vi "ConvertPB_AOupdates.vi"(0 "PB VLIW Array in":T2(array[cluster]) {"Output Bits" format="%x"}, 1 "Definitions":T1={"External MemorySize"=32768, "Internal Memory Size"=512, "Overhead Ticks"=3, "Min Delay Loops"=3, "Loop Count Correction"=1, "Long Delay Loop Count Correction"=2, "Min Instruction Ticks"=6, "Long Delay Ticks"=4294967295, "Clock Period (s)"=1e-08, "Overhead Time (s)"=3e-08, "Min Instruction Cycle Time (s)"=9e-08, "Long Delay Time (s) "=42.94967298} {"Long Delay Time (s)" format="%.8p"; "Min Instruction Cycle Time (s)" format="%.0p"; "Overhead Time (s)" format="%.0p"; "Clock Period (s)" format="%.0p"; "Long Delay Ticks" format="%.0x"}, 2 "error in (no error)":errorcluster, 3 "Full trigger mask":u32 format="%x") -> (5 "PB VLIW Array out":T2(array[cluster]) {"Output Bits" format="%x"}, 6 "error out":errorcluster)   [LabVIEW 2013, in "PulseBlaster.lvlib"]
doc: "Convert AO updates to two pulses to allow consecutive AO pulses. Replicates the whole PB sequence execpt for channel 22 (AO tigger) and the PB halt channel."
uses:
  PulseBlaster.lvlib
panel:
  in  "BeginLoop pointer":u32
  # "(Period*Long D Ticks)+Overhead time"
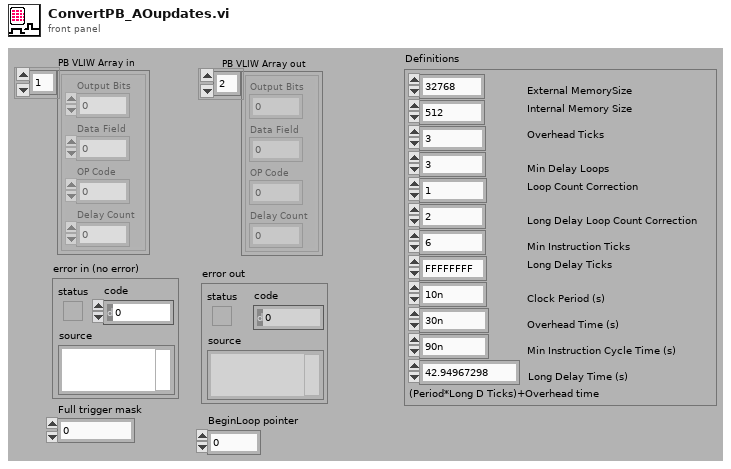
[diagram p1: front panel]
types:
  T1 = cluster{"External MemorySize":u16, "Internal Memory Size":u16, "Overhead Ticks":u8, "Min Delay Loops":u8, "Loop Count Correction":u8, "Long Delay Loop Count Correction":u8, "Min Instruction Ticks":u8, "Long Delay Ticks":u64, "Clock Period (s)":dbl, "Overhead Time (s)":dbl, "Min Instruction Cycle Time (s)":dbl, "Long Delay Time (s) ":dbl}
  T2 = cluster{"Output Bits":u32, "Data Field":u32, "OP Code":u8, "Delay Count":u64}[]
  T3 = cluster{"Output Bits":u32, "Data Field":u32, "OP Code":u8, "Delay Count":u32}[]
  T4 = cluster{"Output Bits":u32, "Data Field":u32, "OP Code":u8, "Delay Count":u64}
  T5 = cluster{"Output Bits":u32, "Data Field":u32, "OP Code":i32, "Delay Count":u64}[]
  T6 = cluster{"Output Bits":u32, "Data Field":u32, "OP Code":u8, u64}
  T7 = cluster{"Output Bits":u32, "BeginLoop pointer":u32, "OP Code":u8, "Delay Count":u64}
  T8 = cluster{"Output Bits":u32, "BeginLoop pointer":u32, "OP Code":i32, "Delay Count":u64}[]
  T9 = cluster{u32, "BeginLoop pointer":u32, "OP Code":u8, u64}
  T10 = cluster{"Output Bits":u32, "Data Field":u32, i32, u64}
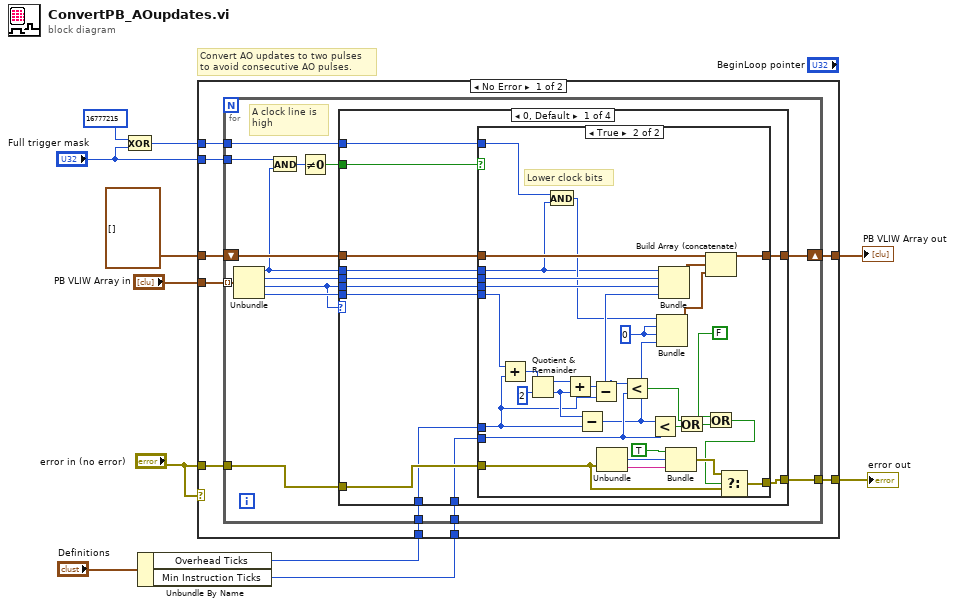
[diagram p0: block diagram]
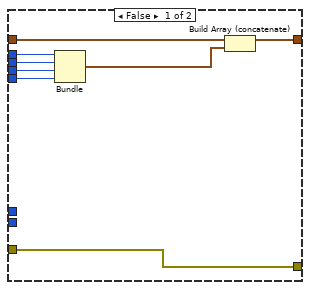
[diagram p2: hidden frame]
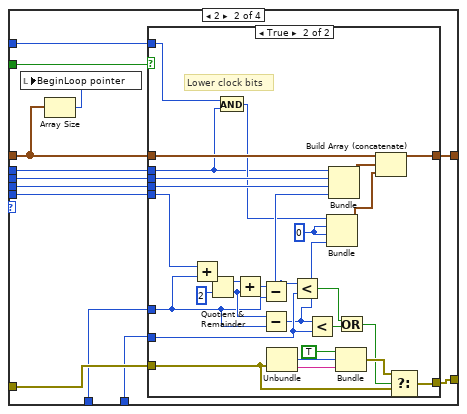
[diagram p3: hidden frame]
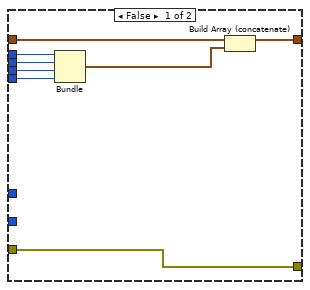
[diagram p4: hidden frame]
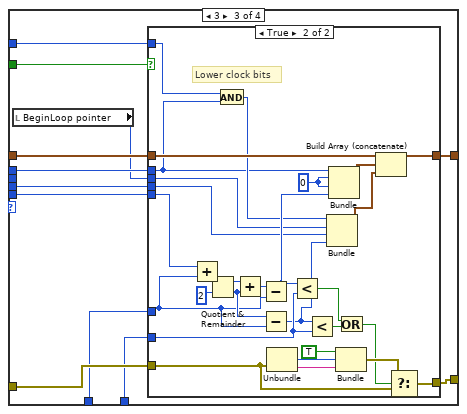
[diagram p5: hidden frame]
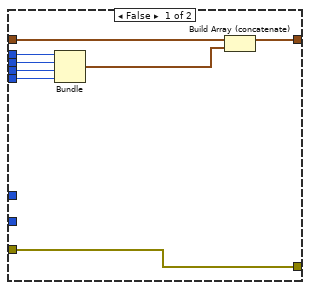
[diagram p6: hidden frame]
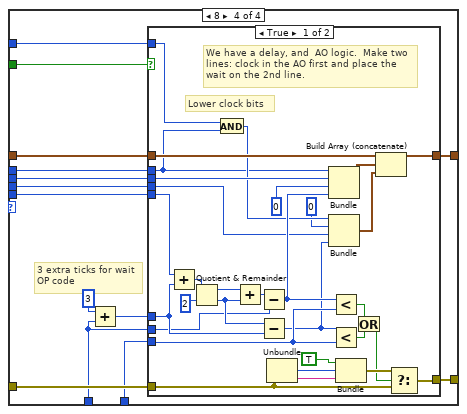
[diagram p7: hidden frame]
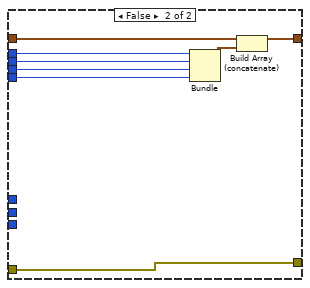
[diagram p8: hidden frame]
diagram:
  # "Convert AO updates to two pulses\nto avoid consecutive AO pulses."
  n1 = Exclusive Or(1:"Full trigger mask", 2:u32 16777215) -> (0:w4:u32)
  n2 = Unbundle By Name("Definitions") -> ("Overhead Ticks"=w2:u8, "Min Instruction Ticks"=w1:u8)
  n3 = case shown="No Error" "error in (no error)" {
    tunnel: T3 [] -> [w20 _]
    tunnel: [w19 w240] -> w10
    tunnel: w2 -> [w18 _]
    tunnel: w1 -> [w17 _]
    tunnel: "PB VLIW Array in" -> [w16 w240]
    tunnel: "error in (no error)" -> [w15 w239]
    tunnel: [w14 w239] -> w8
    tunnel: "Full trigger mask" -> [w13 _]
    tunnel: w4 -> [w12 _]
    frame No Error {
      n4 = for {
        tunnel: w16 -> [w35] mode=indexing
        shift-right: [w27] -> w19
        shift-left: w20 -> [w32]
        tunnel: w15 -> [w31]
        tunnel: [w30] -> w14
        tunnel: w18 -> [w29]
        tunnel: w17 -> [w28]
        tunnel: w13 -> [w22]
        tunnel: w12 -> [w21]
        # "A clock line is \nhigh"
        n5 = Unbundle(w35) -> ("Output Bits"=w25:u32, "Data Field"=w34:u32, "OP Code"=w26:u8, "Delay Count"=w33:u64)
        n6 = And(x=w22, y=w25) -> (x .and. y?=w24:u32)
        n7 = Not Equal To 0?(x=w24) -> (x != 0?=w23:bool)
        n8 = case shown="0, Default" w26 {
          tunnel: w34 -> [w47 w99 _ w199]
          tunnel: w26 -> [w46 w98 w148 w198]
          tunnel: w33 -> [w45 w97 w147 w197]
          tunnel: w32 -> [w44 w89 w140 w196]
          tunnel: w31 -> [w43 w96 w146 w195]
          tunnel: [w42 w95 w145 w194] -> w30
          tunnel: w29 -> [w41 w94 w144 w187]
          tunnel: w28 -> [w40 w93 w143 w193]
          tunnel: w25 -> [w39 w92 w142 w192]
          tunnel: [w38 w91 w141 w191] -> w27
          tunnel: w23 -> [w37 w88 w138 w190]
          tunnel: w21 -> [w36 w87 w137 w186]
          frame 0, Default {
            n9 = case shown="True" w37 {
              tunnel: w39 -> [w55 w57]
              tunnel: w47 -> [w54 w76]
              tunnel: w46 -> [w53 w65]
              tunnel: w45 -> [w52 w86]
              tunnel: [w50 w79] -> w38
              tunnel: w44 -> [w49 w78]
              tunnel: [w48 w71] -> w42
              tunnel: w43 -> [w48 w70]
              tunnel: w41 -> [_ w69]
              tunnel: w40 -> [_ w68]
              tunnel: w36 -> [_ w56]
              frame False {
                n10 = Bundle("Output Bits"=w55, "Data Field"=w54, "OP Code"=w53, "Delay Count"=w52) -> (w51:T4)  [unwired: 1 out]
                n11 = Build Array (concatenate)(w49, w51) -> (w50:T5)
              }
              frame True {
                w58 = 0
                # "Lower clock bits"
                n12 = Add(x=w86, y=w69) -> (x+y=w85:u64)
                n13 = Quotient & Remainder(x=w85, y=u32 2) -> (x-y*floor(x/y)=w83:u64, floor(x/y)=w81:u64)
                n14 = And(x=w56, y=w57) -> (x .and. y?=w64:u32)
                n15 = Add(x=w83, y=w81) -> (x+y=w82:u64)
                n16 = Subtract(x=w81, y=w69) -> (x-y=w66:u64)
                n17 = Subtract(x=w82, y=w69) -> (x-y=w77:u64)
                n18 = Unbundle(w70) -> ("code"=w73:i32, "source"=w74:string)  [unwired: 1 out]
                n19 = Less?(x=w77, y=w68) -> (x < y?=w80:bool)
                n20 = Less?(x=w66, y=w68) -> (x < y?=w67:bool)
                n21 = Bundle(w64, w58, w58, w66) -> (w59:cluster{u32, i32, i32, u64})  [unwired: 1 out]
                n22 = Bundle("Output Bits"=w57, "Data Field"=w76, "OP Code"=w65, w77) -> (w60:T6)  [unwired: 1 out]
                n23 = Bundle(TRUE, "code"=w73, "source"=w74) -> (w72:cluster{bool, "code":i32, "source":string})  [unwired: 1 out]
                n24 = Or(x=w80, y=w67) -> (x .or. y?=w61:bool)
                n25 = Build Array (concatenate)(w78, w60, w59) -> (w79:T5)
                n26 = Or(x=FALSE, y=w61) -> (x .or. y?=w62:bool)
                n27 = Select(t=w72, s=w62, f=w70) -> (s? t:f=w71:errorcluster)
              }
            }
          }
          frame 2 {
            n28 = Array Size(array=w89) -> (size(s)=w90:i32)
            n29 = local write "BeginLoop pointer"(w90) -> ()
            n30 = case shown="True" w88 {
              tunnel: w92 -> [w107 w109]
              tunnel: w99 -> [w106 w126]
              tunnel: w98 -> [w105 w115]
              tunnel: w97 -> [w104 w136]
              tunnel: [w102 w129] -> w91
              tunnel: w89 -> [w101 w128]
              tunnel: [w100 w121] -> w95
              tunnel: w96 -> [w100 w120]
              tunnel: w94 -> [_ w119]
              tunnel: w93 -> [_ w118]
              tunnel: w87 -> [_ w108]
              frame False {
                n31 = Bundle("Output Bits"=w107, "Data Field"=w106, "OP Code"=w105, "Delay Count"=w104) -> (w103:T4)  [unwired: 1 out]
                n32 = Build Array (concatenate)(w101, w103) -> (w102:T5)
              }
              frame True {
                w111 = 0
                # "Lower clock bits"
                n33 = Add(x=w136, y=w119) -> (x+y=w135:u64)
                n34 = Quotient & Remainder(x=w135, y=u32 2) -> (x-y*floor(x/y)=w133:u64, floor(x/y)=w131:u64)
                n35 = And(x=w108, y=w109) -> (x .and. y?=w114:u32)
                n36 = Add(x=w133, y=w131) -> (x+y=w132:u64)
                n37 = Subtract(x=w132, y=w119) -> (x-y=w127:u64)
                n38 = Subtract(x=w131, y=w119) -> (x-y=w116:u64)
                n39 = Unbundle(w120) -> ("code"=w123:i32, "source"=w124:string)  [unwired: 1 out]
                n40 = Less?(x=w127, y=w118) -> (x < y?=w130:bool)
                n41 = Less?(x=w116, y=w118) -> (x < y?=w117:bool)
                n42 = Bundle(w114, w111, w111, w116) -> (w112:cluster{u32, i32, i32, u64})  [unwired: 1 out]
                n43 = Bundle("Output Bits"=w109, "Data Field"=w126, "OP Code"=w115, w127) -> (w113:T6)  [unwired: 1 out]
                n44 = Bundle(TRUE, "code"=w123, "source"=w124) -> (w122:cluster{bool, "code":i32, "source":string})  [unwired: 1 out]
                n45 = Or(x=w130, y=w117) -> (x .or. y?=w110:bool)
                n46 = Build Array (concatenate)(w128, w113, w112) -> (w129:T5)
                n47 = Select(t=w122, s=w110, f=w120) -> (s? t:f=w121:errorcluster)
              }
            }
          }
          frame 3 {
            n48 = local read "BeginLoop pointer"() -> (w139:u32)
            n49 = case shown="True" w138 {
              tunnel: w142 -> [w156 w158]
              tunnel: w139 -> [w155 w175]
              tunnel: w148 -> [w154 w164]
              tunnel: w147 -> [w153 w185]
              tunnel: [w151 w178] -> w141
              tunnel: w140 -> [w150 w177]
              tunnel: [w149 w170] -> w145
              tunnel: w146 -> [w149 w169]
              tunnel: w144 -> [_ w168]
              tunnel: w143 -> [_ w167]
              tunnel: w137 -> [_ w157]
              frame False {
                n50 = Bundle("Output Bits"=w156, "BeginLoop pointer"=w155, "OP Code"=w154, "Delay Count"=w153) -> (w152:T7)  [unwired: 1 out]
                n51 = Build Array (concatenate)(w150, w152) -> (w151:T8)
              }
              frame True {
                w160 = 0
                # "Lower clock bits"
                n52 = Add(x=w185, y=w168) -> (x+y=w184:u64)
                n53 = Quotient & Remainder(x=w184, y=u32 2) -> (x-y*floor(x/y)=w182:u64, floor(x/y)=w180:u64)
                n54 = And(x=w157, y=w158) -> (x .and. y?=w163:u32)
                n55 = Add(x=w182, y=w180) -> (x+y=w181:u64)
                n56 = Subtract(x=w181, y=w168) -> (x-y=w176:u64)
                n57 = Subtract(x=w180, y=w168) -> (x-y=w165:u64)
                n58 = Unbundle(w169) -> ("code"=w172:i32, "source"=w173:string)  [unwired: 1 out]
                n59 = Less?(x=w176, y=w167) -> (x < y?=w179:bool)
                n60 = Less?(x=w165, y=w167) -> (x < y?=w166:bool)
                n61 = Bundle(w163, "BeginLoop pointer"=w175, "OP Code"=w164, w165) -> (w161:T9)  [unwired: 1 out]
                n62 = Bundle("Output Bits"=w158, w160, w160, w176) -> (w162:cluster{"Output Bits":u32, i32, i32, u64})  [unwired: 1 out]
                n63 = Bundle(TRUE, "code"=w172, "source"=w173) -> (w171:cluster{bool, "code":i32, "source":string})  [unwired: 1 out]
                n64 = Or(x=w179, y=w166) -> (x .or. y?=w159:bool)
                n65 = Build Array (concatenate)(w177, w162, w161) -> (w178:T8)
                n66 = Select(t=w171, s=w159, f=w169) -> (s? t:f=w170:errorcluster)
              }
            }
          }
          frame 8 {
            # "3 extra ticks for wait\nOP code"
            n67 = Add(x=u8 3, y=w187) -> (x+y=w188:u8)
            n68 = case shown="True" w190 {
              tunnel: w192 -> [w201 w233]
              tunnel: w199 -> [w220 w236]
              tunnel: w198 -> [w204 w235]
              tunnel: w197 -> [w230 w232]
              tunnel: [w223 w238] -> w191
              tunnel: w196 -> [w222 w237]
              tunnel: [w215 w231] -> w194
              tunnel: w195 -> [w214 w231]
              tunnel: w188 -> [w213 _]
              tunnel: w193 -> [w212 _]
              tunnel: w187 -> [w202 _]
              tunnel: w186 -> [w200 _]
              frame True {
                # "We have a delay, and  AO logic.  Make two  lines: clock in the AO first and place the wait on the 2nd line."
                # "Lower clock bits"
                n69 = Add(x=w230, y=w213) -> (x+y=w229:u64)
                n70 = Quotient & Remainder(x=w229, y=u32 2) -> (x-y*floor(x/y)=w227:u64, floor(x/y)=w225:u64)
                n71 = And(x=w200, y=w201) -> (x .and. y?=w209:u32)
                n72 = Add(x=w227, y=w225) -> (x+y=w226:u64)
                n73 = Subtract(x=w226, y=w202) -> (x-y=w221:u64)
                n74 = Subtract(x=w225, y=w213) -> (x-y=w210:u64)
                n75 = Unbundle(w214) -> ("code"=w217:i32, "source"=w218:string)  [unwired: 1 out]
                n76 = Bundle("Output Bits"=w201, "Data Field"=w220, 0, w221) -> (w208:T10)  [unwired: 1 out]
                n77 = Bundle(w209, 0, "OP Code"=w204, w210) -> (w207:cluster{u32, i32, "OP Code":u8, u64})  [unwired: 1 out]
                n78 = Less?(x=w221, y=w212) -> (x < y?=w224:bool)
                n79 = Less?(x=w210, y=w212) -> (x < y?=w211:bool)
                n80 = Bundle(TRUE, "code"=w217, "source"=w218) -> (w216:cluster{bool, "code":i32, "source":string})  [unwired: 1 out]
                n81 = Or(x=w224, y=w211) -> (x .or. y?=w203:bool)
                n82 = Build Array (concatenate)(w222, w208, w207) -> (w223:T5)
                n83 = Select(t=w216, s=w203, f=w214) -> (s? t:f=w215:errorcluster)
              }
              frame False {
                n84 = Bundle("Output Bits"=w233, "Data Field"=w236, "OP Code"=w235, "Delay Count"=w232) -> (w234:T4)  [unwired: 1 out]
                n85 = Build Array (concatenate)(w237, w234) -> (w238:T5)
              }
            }
          }
        }
      }
    }
    frame Error {
    }
  }
  "error out" <- w8
  "PB VLIW Array out" <- w10
